vi "arm safety.vi"(8 "Min Rate":dbl, 9 "Reverse Limit":dbl, 10 "Forward Limit":dbl, 11 "Desired Rate":dbl) -> (0 "Input Out of Range":bool, 1 "Encoder Directional Issue":bool, 2 "At Distance Limit":bool, 3 "Output Rate":dbl, 4 "Encoder Failure":bool)   [LabVIEW 2014]
uses:
  global variables/devrefs.vi
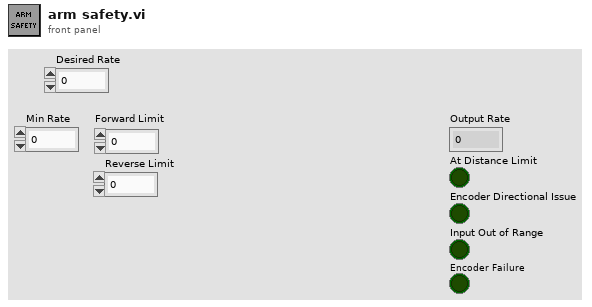
[diagram p1: front panel]
types:
  T1 = typedef "WPI_EncoderDevRef.ctl" = cluster{"DevStatus":errorcluster, "EncoderIndex":T2, "CounterIndex":T3, "DistancePerCount":dbl, "Decoding Type":T4}
  T2 = typedef "FPGA_EncoderIdx.ctl" = enum8{"Enc 0", "Enc 1", "Enc 2", "Enc 3", "Enc 4", "Enc 5", "Enc 6", "Enc 7", "Invalid"}
  T3 = typedef "FPGA_CounterCtrSystemIndex.ctl" = enum8{"Ctr 0", "Ctr 1", "Ctr 2", "Ctr 3", "Ctr 4", "Ctr 5", "Ctr 6", "Ctr 7", "Invalid"}
  T4 = typedef "WPI_EncoderType.ctl" = enum16{"1x", "2x", "4x"}
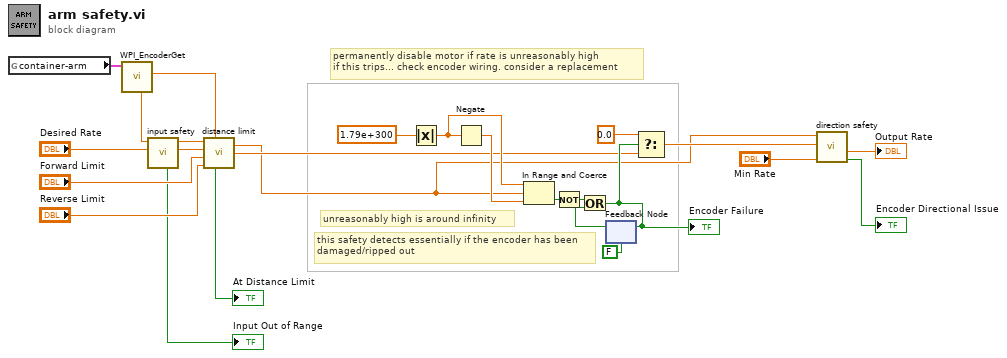
[diagram p0: block diagram]
diagram:
  # "this safety detects essentially if the encoder has been\ndamaged/ripped out"
  # "unreasonably high is around infinity"
  # "permanently disable motor if rate is unreasonably high\nif this trips... check encoder wiring. consider a replacement"
  n1 = global read "devrefs.vi" "container-arm"() -> (w9:T1)
  n2 = call <vilib>:"WPI_EncoderGet.vi"("EncoderDevRef"=w9) -> ("Distance"=w7:dbl, "Rate"=w8:dbl)  [unwired: 5 in, 4 out]
  n3 = call "input safety.vi"("Desired Rate"="Desired Rate", "Encoder Rate"=w8) -> ("Safe Rate"=w25:dbl, "Encoder Rate Out"=w24:dbl, "Input Out of Range"=→"Input Out of Range":bool)  [unwired: 7 in]
  n4 = call "distance limit.vi"("Encoder Rate"=w24, "Encoder Distance"=w7, "Desired Rate"=w25, "Forward Limit"="Forward Limit", "Reverse Limit"="Reverse Limit") -> ("At Distance Limit"=→"At Distance Limit":bool, "Encoder Rate Out"=w12:dbl, "Output Rate"=w14:dbl)  [unwired: 1 in]
  n5 = Absolute Value(x=1.79e+300 ("Max Rate")) -> (abs(x)=w15:dbl)
  n6 = Negate(x=w15) -> (-x=w17:dbl)
  n7 = In Range and Coerce(upper limit=w15, x=w12, lower limit=w17) -> (In Range?=w19:bool)  [unwired: 1 out]
  n8 = Not(x=w19) -> (.not. x?=w18:bool)
  n9 = feedback #1(FALSE ("x > y?")) -> (w20:bool)
  n10 = Or(x=w18, y=w20) -> (x .or. y?=w23:bool)
  "Encoder Failure" <- w23
  n11 = feedback-in #1(w23) -> ()
  n12 = Select(t=0.0, s=w23, f=w14) -> (s? t:f=w13:dbl)
  n13 = call "direction safety.vi"("Min Rate"="Min Rate", "Desired Rate"=w13, "Encoder Rate"=w12) -> ("Encoder Directional Issue"=→"Encoder Directional Issue":bool, "Super Safe Rate"=→"Output Rate":dbl)  [unwired: 2 in, 1 out]
